vi "openCam.vi"(8 "error in (no error)":errorcluster, 10 "Camera Opened":bool, 11 "Boolean in":refnum<vi>) -> (0 "error out":errorcluster, 2 "Ydim":u32, 3 "Xdim":u32)   [LabVIEW 2015]
uses:
  Public/Documents/SItoolkit/LabVIEW/Examples2015_6_0_2_9/Fast Examples/Open-Close Hardware/CamHandle.vi
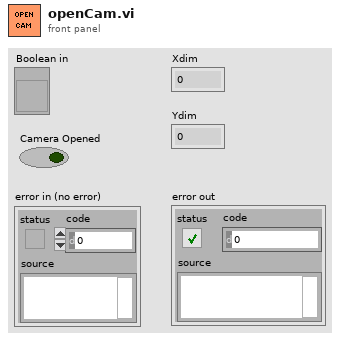
[diagram p1: front panel]
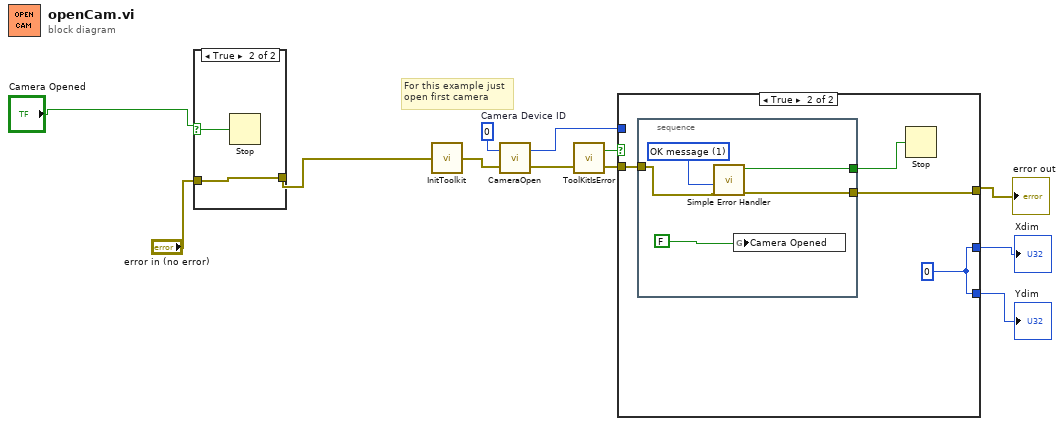
[diagram p0: block diagram]
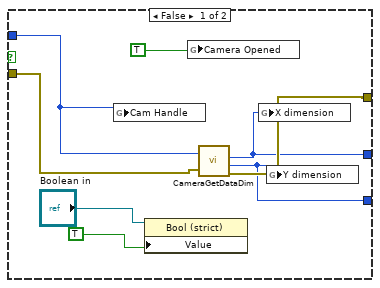
[diagram p3: hidden frame]
diagram:
  w5 = u32 0  # Camera Device ID
  # "For this example just\nopen first camera"
  n1 = case shown="True" "Camera Opened" {
    selector: "Camera Opened" -> [_ w14]
    tunnel: [w13 w15] -> w10
    tunnel: "error in (no error)" -> [w13 w15]
    frame False {
    }
    frame True {
      n2 = Stop(stop? (T)=w14) -> ()
    }
  }
  n3 = call <userlib>:"InitToolkit.vi"("error in"=w10) -> ("error out"=w1:errorcluster)
  n4 = call <userlib>:"CameraOpen.vi"("error in"=w1, "Camera Device ID"=w5) -> ("error out"=w2:errorcluster, "Camera Handle"=w6:u32)
  n5 = call <userlib>:"ToolKitIsError.vi"("error in"=w2) -> ("error out"=w4:errorcluster, "Error Flag"=w3:bool)  [unwired: 1 in]
  n6 = case shown="True" w3 {
    tunnel: w4 -> [w22 w27]
    tunnel: [w21 w26] -> w7
    tunnel: w6 -> [w23 _]
    tunnel: [w17 w24] -> w11
    tunnel: [w16 w24] -> w12
    frame False {
      n7 = global write "CamHandle.vi" "Cam Handle"(w23) -> ()
      n8 = property class="Bool (strict)"(reference="Boolean in", "Value"=TRUE) -> ()  [unwired: 1 in, 2 out]
      n9 = global write "CamHandle.vi" "Camera Opened"(TRUE) -> ()
      n10 = call <userlib>:"CameraGetDataDim.vi"("Camera Handle"=w23, "error in"=w22) -> ("Xdim"=w17:u32, "Ydim"=w16:u32, "error out"=w21:errorcluster)  [unwired: 1 out]
      n11 = global write "CamHandle.vi" "X dimension"(w17) -> ()
      n12 = global write "CamHandle.vi" "Y dimension"(w16) -> ()
    }
    frame True {
      w24 = 0
      n13 = stacked-sequence {
        tunnel: w27 -> [w31]
        tunnel: [w30] -> w25
        tunnel: [w29] -> w26
        frame #0 {
          w32 = u16 1 items=["no dialog", "OK message", "continue or stop message"] ("type of dialog (OK msg:1)")
          n14 = call <vilib>:"Simple Error Handler.vi"("type of dialog (OK msg:1)"=w32, "error in (no error)"=w31) -> ("error?"=w30:bool, "error out"=w29:errorcluster)  [unwired: 3 in, 3 out]
          n15 = global write "CamHandle.vi" "Camera Opened"(FALSE) -> ()
        }
      }
      n16 = Stop(stop? (T)=w25) -> ()
    }
  }
  "Ydim" <- w12
  "Xdim" <- w11
  "error out" <- w7
